vi "External_Retain Wire Values.vi"(8 "error in":errorcluster, 9 "Retain Wire Values":bool, 10 "Selected VIs":string[](array[string]), 11 "Application in":refnum<vi>) -> (0 "error out":errorcluster)   [LabVIEW 2013]
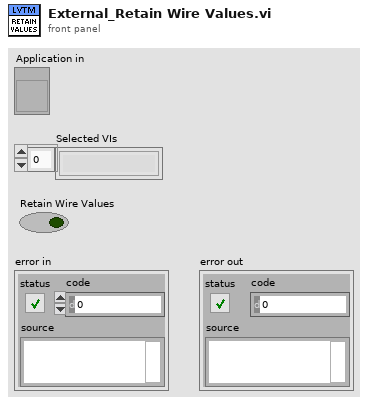
[diagram p1: front panel]
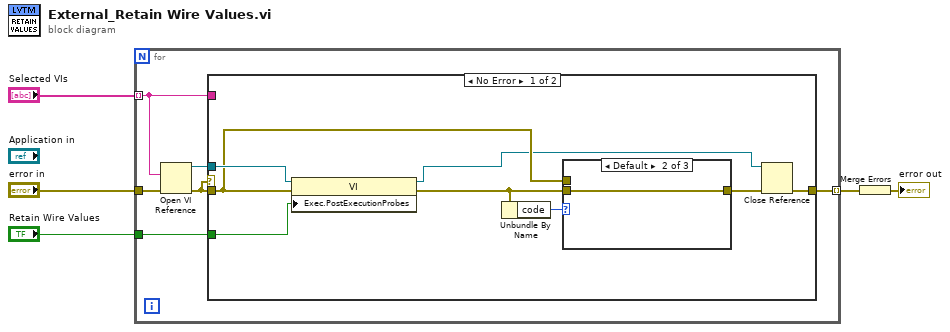
[diagram p0: block diagram]
diagram:
  n1 = for {
    tunnel: "Selected VIs" -> [w8] mode=indexing
    tunnel: "error in" -> [w10]
    tunnel: [w9] -> w1 mode=indexing
    tunnel: "Retain Wire Values" -> [w7]
    n2 = Open VI Reference(vi path=w8, error in (no error)=w10) -> (vi reference=w11:refnum<vi>, error out=w6:errorcluster)  [unwired: 4 out]
    n3 = case shown="No Error" w6 {
      tunnel: w11 -> [w19 _]
      tunnel: [w18 _] -> w9
      tunnel: w8 -> [_ _]
      tunnel: w6 -> [w14 _]
      tunnel: w7 -> [w12 _]
      frame No Error {
        n4 = property class="VI"(reference=w19, error in=w14, "Exec.PostExecutionProbes"=w12) -> (reference out=w13:refnum<vi>, error out=w15:errorcluster)
        n5 = Unbundle By Name(w15) -> ("code"=w17:i32)
        n6 = case shown="Default" w17 {
          tunnel: [w20 w21 w22] -> w16
          tunnel: w15 -> [w20 w21 _]
          tunnel: w14 -> [_ _ w22]
          frame 0 {
          }
          frame Default {
          }
          frame 1035 {
            # "Operation is invalid for this type of VI.\nIgnore Error."
          }
        }
        n7 = Close Reference(reference=w13, error in (no error)=w16) -> (error out=w18:errorcluster)
      }
      frame Error {
        # "This VI is no longer in the memory"
      }
    }
  }
  n8 = Merge Errors(w1) -> (→"error out":errorcluster)
